vi "EVAL-AD5764EB Example.vi"() -> ()   [LabVIEW 2018]
uses:
  EVAL-AD5764EB.lvlib
panel:
  in  "VISA resource name":refnum<visa-resource-name>
  in  "Ch D":dbl(knob) scale=-10.0..10.0
  in  "Ch C":dbl(knob) scale=-10.0..10.0
  in  "Ch B":dbl(knob) scale=-10.0..10.0
  in  "Ch A":dbl(knob) scale=-10.0..10.0
  in  "stop":bool
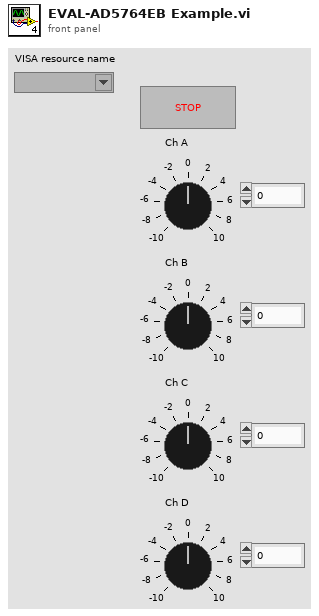
[diagram p1: front panel]
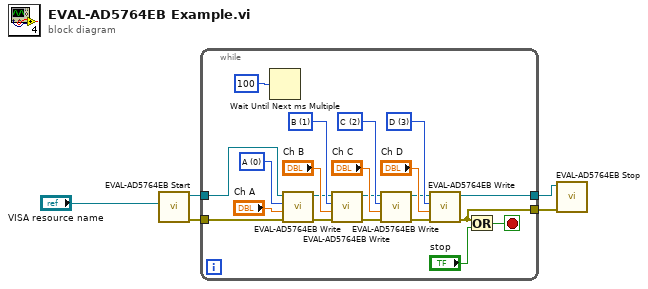
[diagram p0: block diagram]
diagram:
  n1 = call "EVAL-AD5764EB Start.vi"("VISA resource name"="VISA resource name") -> ("error out"=w4:errorcluster, "VISA resource name out"=w3:refnum<visa-resource-name>)  [unwired: 9 in]
  n2 = while {
    tunnel: w4 -> [w24]
    tunnel: w3 -> [w23]
    tunnel: [w10] -> w2
    tunnel: [w9] -> w1
    stop <- w8 stop-if-true
    w14 = u16 3 items=["A", "B", "C", "D"] ("Chanel")
    w15 = u16 2 items=["A", "B", "C", "D"] ("Chanel")
    w16 = u16 1 items=["A", "B", "C", "D"] ("Chanel")
    w25 = u16 0 items=["A", "B", "C", "D"] ("Chanel")
    n3 = Wait Until Next ms Multiple(millisecond multiple=u32 100) -> ()  [unwired: 1 out]
    n4 = call "EVAL-AD5764EB Write.vi"("error in (no error)"=w24, "Voltage"="Ch A", "Chanel"=w25, "VISA resource name"=w23) -> ("error out"=w19:errorcluster, "VISA resource name out"=w13:refnum<visa-resource-name>)  [unwired: 6 in]
    n5 = call "EVAL-AD5764EB Write.vi"("error in (no error)"=w19, "Voltage"="Ch B", "Chanel"=w16, "VISA resource name"=w13) -> ("error out"=w18:errorcluster, "VISA resource name out"=w12:refnum<visa-resource-name>)  [unwired: 6 in]
    n6 = call "EVAL-AD5764EB Write.vi"("error in (no error)"=w18, "Voltage"="Ch C", "Chanel"=w15, "VISA resource name"=w12) -> ("error out"=w17:errorcluster, "VISA resource name out"=w11:refnum<visa-resource-name>)  [unwired: 6 in]
    n7 = call "EVAL-AD5764EB Write.vi"("error in (no error)"=w17, "Voltage"="Ch D", "Chanel"=w14, "VISA resource name"=w11) -> ("error out"=w9:errorcluster, "VISA resource name out"=w10:refnum<visa-resource-name>)  [unwired: 6 in]
    n8 = Or(x=w9, y="stop") -> (x .or. y?=w8:bool)
  }
  n9 = call "EVAL-AD5764EB Stop.vi"("error in (no error)"=w1, "VISA resource name"=w2) -> ()  [unwired: 9 in, 1 out]
